vi "GetFirstProcessModule_EventRef.vi"(8 "error in (no error)":errorcluster, 9 "data":T1, 11 "Qbus in":refnum<class "Qbus.lvclass">) -> (0 "error out":errorcluster, 3 "Qbus out":refnum<class "Qbus.lvclass">)   [LabVIEW 2017, in "FileFlow.lvlib"]
doc: "Sends an in-memory TDMS file to the first process in the Fileflow Script via a Qbus message. The first process operates on the file, and then transfers it to the next process."
uses:
  <vilib>/addons/InsightCM/Devices/Shared/Common/FileFlow/FileFlow.lvlib
  <vilib>/addons/Qbus/Qbus.lvclass
  <vilib>/addons/InsightCM/Devices/Shared/Common/FileFlow/controls/data_eventRef.ctl
  <vilib>/addons/InsightCM/Devices/Shared/Common/DataEvent/controls/EventReference.ctl
  <vilib>/addons/InsightCM/Devices/Shared/Common/DataEvent/controls/Event.ctl
  <vilib>/addons/InsightCM/MessageBus/Base/controls/DataEvent.ctl
  <vilib>/addons/InsightCM/MessageBus/Base/controls/KeyValuePair.ctl
  <vilib>/addons/InsightCM/Devices/Shared/Common/DataEvent/controls/DataSet.ctl
  <vilib>/addons/InsightCM/MessageBus/Base/controls/DataSetMetadata.ctl
  <vilib>/addons/InsightCM/MessageBus/Base/controls/TrendPoint.ctl
  <vilib>/addons/InsightCM/MessageBus/Base/controls/TrendAlarmUpdate.ctl
  <vilib>/addons/InsightCM/MessageBus/Base/controls/TrendAlarmTransition.ctl
  <vilib>/addons/PointValueMap/controls/PointMap.ctl
  <vilib>/addons/PointValueMap/PointValueMap.lvlib
  <vilib>/addons/InsightCM/Devices/Shared/Common/DataEvent/DataEvent.lvlib
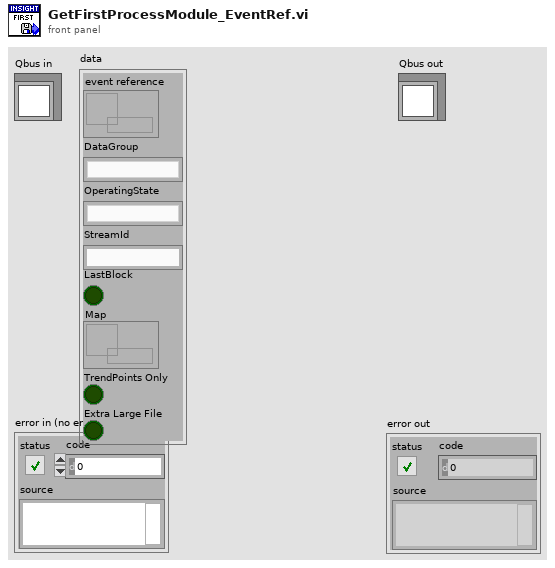
[diagram p1: front panel]
types:
  T1 = typedef "FileFlow.lvlib/data_eventRef.ctl" = cluster{"event reference":T2, "DataGroup":string, "OperatingState":string, "StreamId":string, "LastBlock":bool, "Map":T3, "TrendPoints Only":bool, "Extra Large File":bool}
  T2 = typedef "DataEvent.lvlib/EventReference.ctl" = refnum<data-value>
  T3 = typedef "PointValueMap.lvlib/PointMap.ctl" = refnum<data-value>
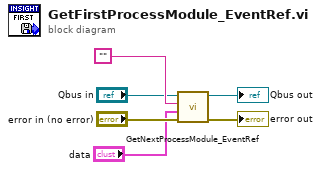
[diagram p0: block diagram]
diagram:
  n1 = call <vilib>:"GetNextProcessModule_EventRef.vi"("error in (no error)"="error in (no error)", "data"="data", "source"="", "Qbus in"="Qbus in") -> ("error out"=→"error out":errorcluster, "Qbus out"=→"Qbus out":refnum<class "Qbus.lvclass">)  [unwired: 6 in]
